vi "CalcForce.vi"(0 "Trap 1X V":waveform(dbl), 1 "T1 alphaX (nm/V)":dbl, 2 "T1 kappaX (pN/nm)":dbl, 3 "T1 offset X":dbl, 7 "Trap 2X V":waveform(dbl), 11 "Calibration":u16, 12 "T2 alphaX (nm/V)":dbl, 13 "T2 kappaX (pN/nm)":dbl, 14 "T2 offsetX":dbl) -> (4 "Force 1X":waveform(dbl), 6 "Force X":waveform(dbl), 8 "Force 2X":waveform(dbl), 10 "BeadDeflection":waveform(dbl), 15 "Out Names":T1)   [LabVIEW 2013]
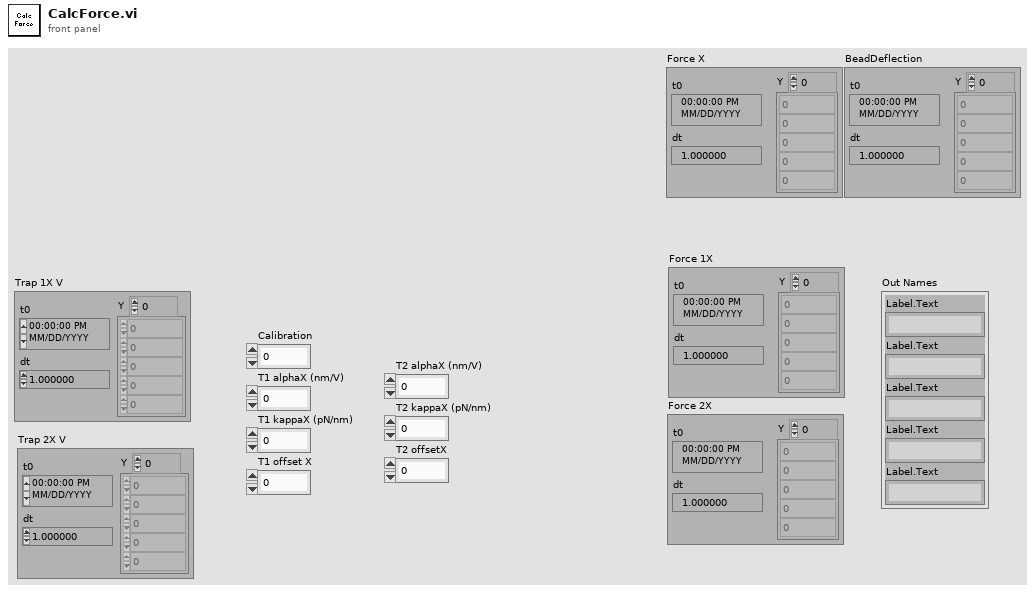
[diagram p1: front panel]
types:
  T1 = cluster{"Label.Text":string, "Label.Text":string, "Label.Text":string, "Label.Text":string, "Label.Text":string}
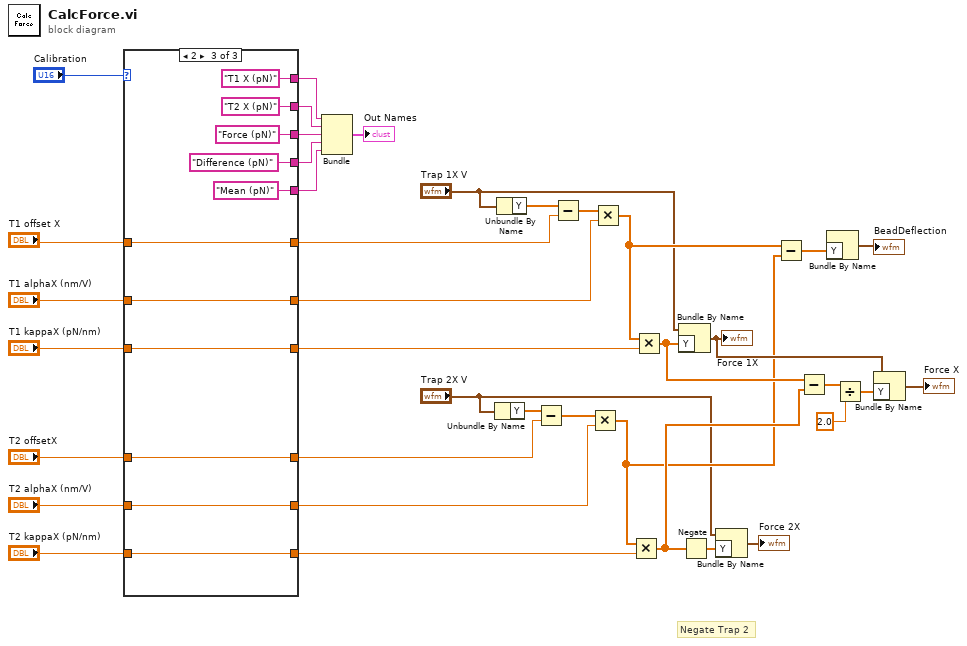
[diagram p0: block diagram]
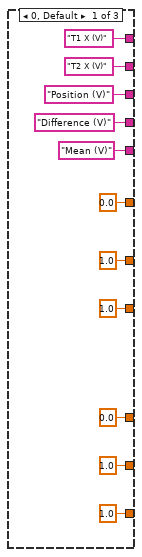
[diagram p2: hidden frame]
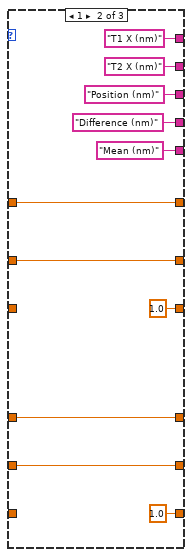
[diagram p3: hidden frame]
diagram:
  # "Negate Trap 2"
  n1 = case shown="2" "Calibration" {
    tunnel: ["T1 X (V)" ("Label.Text") "T1 X (nm)" ("Label.Text") "T1 X (pN)" ("Label.Text")] -> w34
    tunnel: ["T2 X (V)" ("Label.Text") "T2 X (nm)" ("Label.Text") "T2 X (pN)" ("Label.Text")] -> w33
    tunnel: ["Position (V)" ("Label.Text") "Position (nm)" ("Label.Text") "Force (pN)" ("Label.Text")] -> w32
    tunnel: ["Mean (V)" ("Label.Text") "Mean (nm)" ("Label.Text") "Mean (pN)" ("Label.Text")] -> w30
    tunnel: ["Difference (V)" ("Label.Text") "Difference (nm)" ("Label.Text") "Difference (pN)" ("Label.Text")] -> w31
    tunnel: [0.0 ("T1 offset X") w55 w63] -> w26
    tunnel: [1.0 ("T1 alphaX (nm/V)") w54 w62] -> w25
    tunnel: [1.0 ("T1 kappaX (pN/nm)") 1.0 ("T1 kappaX (pN/nm)") w61] -> w24
    tunnel: [0.0 ("T2 offsetX") w50 w64] -> w23
    tunnel: [1.0 ("T2 alphaX (nm/V)") w51 w65] -> w22
    tunnel: [1.0 ("T2 kappaX (pN/nm)") 1.0 ("T2 kappaX (pN/nm)") w66] -> w21
    tunnel: "T2 kappaX (pN/nm)" -> [_ _ w66]
    tunnel: "T2 alphaX (nm/V)" -> [_ w51 w65]
    tunnel: "T2 offsetX" -> [_ w50 w64]
    tunnel: "T1 offset X" -> [_ w55 w63]
    tunnel: "T1 alphaX (nm/V)" -> [_ w54 w62]
    tunnel: "T1 kappaX (pN/nm)" -> [_ _ w61]
    frame 0, Default {
    }
    frame 1 {
    }
    frame 2 {
    }
  }
  n2 = Bundle("Label.Text"=w34, "Label.Text"=w33, "Label.Text"=w32, "Label.Text"=w31, "Label.Text"=w30) -> (→"Out Names":T1)  [unwired: 1 in]
  n3 = Unbundle By Name("Trap 2X V") -> ("Y"=w36:dbl[])
  n4 = Unbundle By Name("Trap 1X V") -> ("Y"=w38:dbl[])
  n5 = Subtract(x=w36, y=w23) -> (x-y=w37:dbl[])
  n6 = Subtract(x=w38, y=w26) -> (x-y=w27:dbl[])
  n7 = Multiply(x=w37, y=w22) -> (x*y=w5:dbl[])
  n8 = Multiply(x=w27, y=w25) -> (x*y=w6:dbl[])
  n9 = Multiply(x=w5, y=w21) -> (x*y=w13:dbl[])
  n10 = Multiply(x=w6, y=w24) -> (x*y=w14:dbl[])
  n11 = Bundle By Name(cluster="Trap 1X V", "Y"=w14) -> (w9:waveform(dbl))
  "Force 1X" <- w9
  n12 = Negate(x=w13) -> (-x=w1:dbl[])
  n13 = Bundle By Name(cluster="Trap 2X V", "Y"=w1) -> (→"Force 2X":waveform(dbl))
  n14 = Subtract(x=w6, y=w5) -> (x-y=w4:dbl[])
  n15 = Subtract(x=w14, y=w13) -> (x-y=w12:dbl[])
  n16 = Bundle By Name("Y"=w4) -> (→"BeadDeflection":waveform(dbl))  [unwired: 1 in]
  n17 = Divide(x=w12, y=2.0) -> (x/y=w10:dbl[])
  n18 = Bundle By Name(cluster=w9, "Y"=w10) -> (→"Force X":waveform(dbl))
